vi "LJstreamUD add data to file.vi"(4 "Scan Rate":dbl=50.0 format="%.2f", 6 "Time":dbl format="%.2f", 9 "Scaled Data":dbl[][](array[numeric]) format="%.3f", 10 "Voltages":dbl[][](array[numeric]) format="%.3f", 11 "file path":path) -> (0 "error":bool)   [LabVIEW 2021]
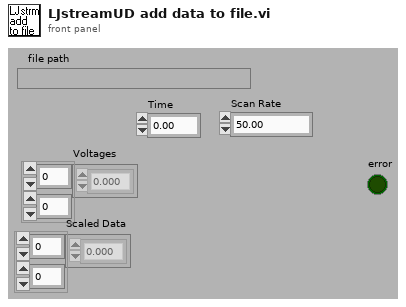
[diagram p1: front panel]
types:
  T1 = enum16{"open", "open or create", "create or replace", "create", "open (read only)"}
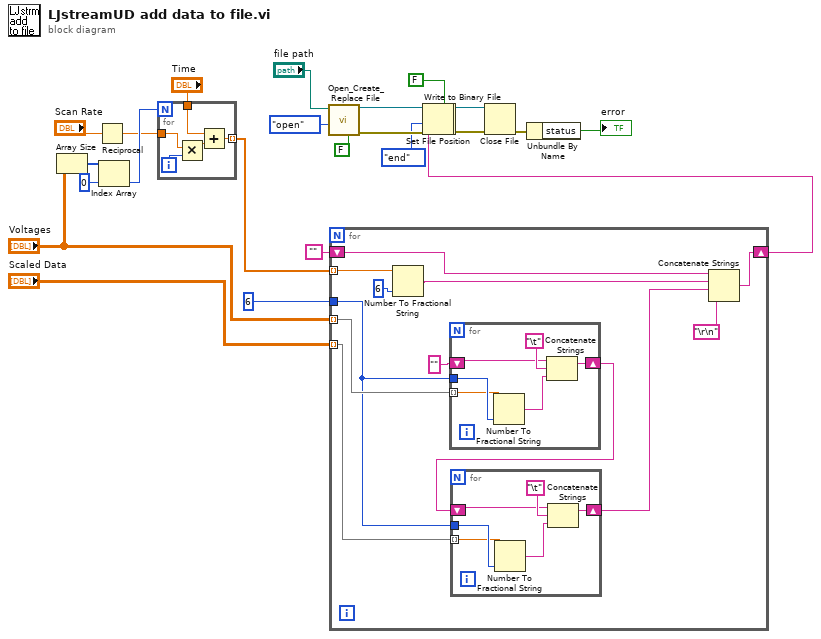
[diagram p0: block diagram]
diagram:
  n1 = Array Size(array="Voltages") -> (size(s)=w15:i32[])
  n2 = Reciprocal(x="Scan Rate") -> (1/x=w10:dbl)
  n3 = Index Array(array=w15, index=0 ("Index")) -> (element=w13:i32)
  n4 = for {
    N: w13 -> [_]
    tunnel: "Time" -> [w30]
    tunnel: w10 -> [w26]
    tunnel: [w29] -> w9 mode=indexing
    i -> [w27]
    n5 = Multiply(x=w26, y=w27) -> (x*y=w28:dbl)
    n6 = Add(x=w30, y=w28) -> (x+y=w29:dbl)
  }
  n7 = call <vilib>:"Open_Create_Replace File.vi"("advisory dialog? (display:T)"=FALSE, "function (open:0)"=T1."open", "file path"="file path") -> ("error out"=w22:errorcluster, "refnum"=w23:refnum<file>)  [unwired: 5 in, 2 out]
  n8 = for {
    shift-right: [w38] -> w6
    shift-left: "" -> [w39]
    tunnel: w9 -> [w41] mode=indexing
    tunnel: "Voltages" -> [w36] mode=indexing
    tunnel: "Scaled Data" -> [w31] mode=indexing
    tunnel: i16 6 ("precision (6)") -> [w32]
    n9 = Number To Fractional String(number=w41, precision (6)=i16 6) -> (F-format string=w40:string)  [unwired: 2 in]
    n10 = for {
      shift-right: [w52] -> w34
      shift-left: "" -> [w53]
      tunnel: w32 -> [w50]
      tunnel: w36 -> [w49] mode=indexing
      n11 = Number To Fractional String(number=w49, precision (6)=w50) -> (F-format string=w51:string)  [unwired: 2 in]
      n12 = Concatenate Strings(w53, "\t", w51) -> (w52:string)
    }
    n13 = for {
      shift-right: [w46] -> w33
      shift-left: w34 -> [w47]
      tunnel: w32 -> [w44]
      tunnel: w31 -> [w43] mode=indexing
      n14 = Number To Fractional String(number=w43, precision (6)=w44) -> (F-format string=w45:string)  [unwired: 2 in]
      n15 = Concatenate Strings(w47, "\t", w45) -> (w46:string)
    }
    n16 = Concatenate Strings(w39, w40, w33, "\r\n") -> (w38:string)
  }
  n17 = Set File Position(refnum=w23, from (0:start)=enum16{"start", "end", "current"}."end" ("pos mode (0:2)"), error in=w22) -> (refnum out=w3:refnum<file>, error out=w2:errorcluster)  [unwired: 1 in]
  n18 = Write to Binary File(file (use dialog)=w3, data=w6, error in=w2, 5:FALSE ("prepend array or string size? (T)")) -> (refnum out=w25:refnum<file>, error out=w24:errorcluster)  [unwired: 2 in, 1 out]
  n19 = Close File(refnum=w25, error in=w24) -> (error out=w17:errorcluster)  [unwired: 1 out]
  n20 = Unbundle By Name(w17) -> ("status"=→"error":bool)
